vi "E05_Estructura_Flat_Sequence.vi"() -> ()   [LabVIEW 2026]
panel:
  out "Boolean1":bool
  out "Boolean3":bool
  out "Boolean2":bool
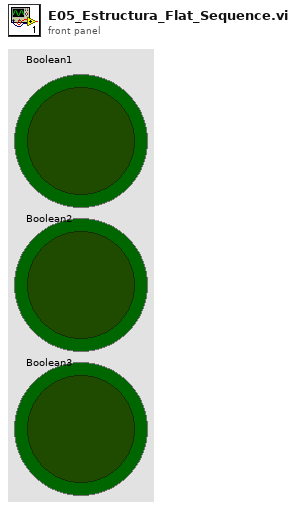
[diagram p1: front panel]
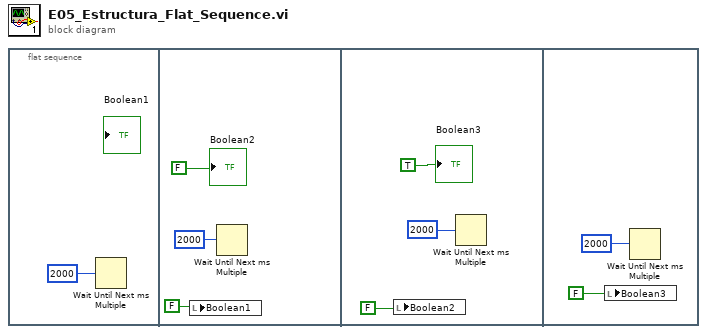
[diagram p0: block diagram]
diagram:
  n1 = flat-sequence {
    frame #0 {
      n2 = Wait Until Next ms Multiple(millisecond multiple=u32 2000) -> ()  [unwired: 1 out]
    }
    frame #1 {
      n3 = local write "Boolean1"(FALSE ("Boolean1")) -> ()
      n4 = Wait Until Next ms Multiple(millisecond multiple=u32 2000) -> ()  [unwired: 1 out]
      "Boolean2" <- FALSE ("Boolean1")
    }
    frame #2 {
      n5 = local write "Boolean2"(FALSE ("Boolean1")) -> ()
      n6 = Wait Until Next ms Multiple(millisecond multiple=u32 2000) -> ()  [unwired: 1 out]
      "Boolean3" <- TRUE
    }
    frame #3 {
      n7 = local write "Boolean3"(FALSE ("Boolean1")) -> ()
      n8 = Wait Until Next ms Multiple(millisecond multiple=u32 2000) -> ()  [unwired: 1 out]
    }
  }
